vi "Get Address Map Element.vi"(2 "niUSRP DSP v2 FPGA":refnum<class "niUSRP Rx DSP v2 FPGA.lvclass">, 5 "index":u8) -> (6 "address map element":T1)   [LabVIEW 2025, in "niUSRP Rx DSP v2 FPGA.lvclass"]
uses:
  niUSRP Rx DSP v2 FPGA.lvclass
  <instrlib>/_niInstr/Instruction Framework/v1/FPGA/Typedefs/Address Map Element.ctl
  <instrlib>/_niInstr/Instruction Framework/v1/FPGA/Typedefs/niInstr Instruction Framework v1 FPGA.lvlib
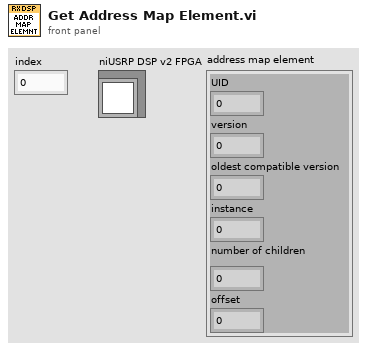
[diagram p1: front panel]
types:
  T1 = typedef "niInstr Instruction Framework v1 FPGA.lvlib/Address Map Element.ctl" = cluster{"UID":u16, "version":u16, "oldest compatible version":u16, "instance":u8, "number of children":u8, "offset":u32}
  T2 = typedef "niInstr Address Space Collection Builder v1 FPGA.lvlib/Parent Metadata.ctl" = cluster{"UID":u16, "version":u16, "oldest compatible version":u16}
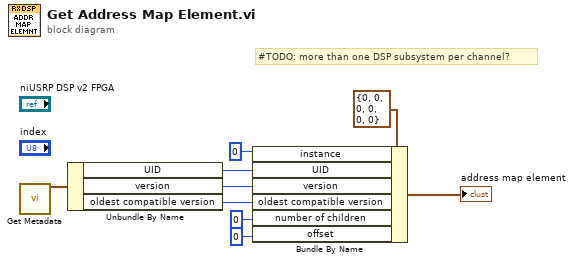
[diagram p0: block diagram]
diagram:
  # "#TODO: more than one DSP subsystem per channel?"
  n1 = call "Get Metadata.vi"() -> ("acq metadata"=w5:T2)  [unwired: 15 in]
  n2 = Unbundle By Name(w5) -> ("UID"=w4:u16, "version"=w3:u16, "oldest compatible version"=w2:u16)
  n3 = Bundle By Name(cluster=T1 {"UID"=0, "version"=0, "oldest compatible version"=0, "instance"=0, "number of children"=0, "offset"=0} ("address map element"), "instance"=u8 0, "UID"=w4, "version"=w3, "oldest compatible version"=w2, "number of children"=u8 0, "offset"=u32 0) -> (→"address map element":T1)
